vi "getDataFileNameInDataPath.vi"(8 "error in (no error)":errorcluster, 10 "FileName":string) -> (0 "error out":errorcluster, 2 "FileNamePathInDataDir":path)   [LabVIEW 2011]
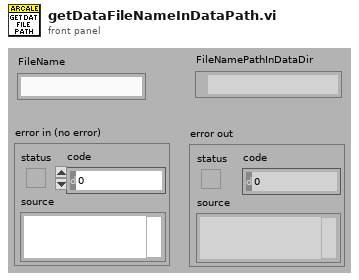
[diagram p1: front panel]
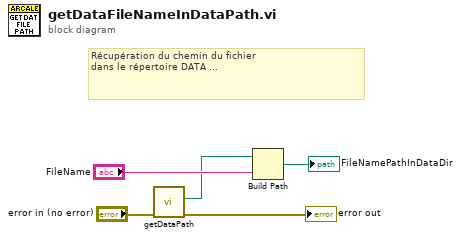
[diagram p0: block diagram]
diagram:
  # "Récupération du chemin du fichier\ndans le répertoire DATA ..."
  n1 = call "getDataPath.vi"("error in (no error)"="error in (no error)") -> ("error out"=→"error out":errorcluster, "DataPath"=w1:path)  [unwired: 9 in]
  n2 = Build Path(base path=w1, name or relative path="FileName") -> (appended path=→"FileNamePathInDataDir":path)
